vi "Write Enable Server Generic UE.vi"(10 "Enable Server Generic UE":bool, 11 "Template Server in":refnum<class "Streamer_server.lvclass">) -> (3 "Template Server out":refnum<class "Streamer_server.lvclass">)   [LabVIEW 2019, in "Streamer_server.lvlib" / "Streamer_server.lvclass"]
doc: "Enable the generic event if you would like to use a single event for capturing all messages. This would be useful if you are planning to implement your own dispatcher logic. \n\nKindly note that enabling the generic event would not generate the individual events."
uses:
  Streamer_server.lvclass
  Streamer_server.lvclass/Streamer_server.ctl
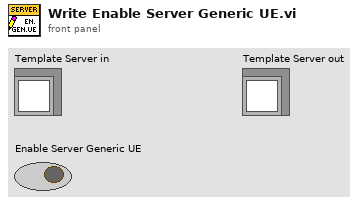
[diagram p1: front panel]
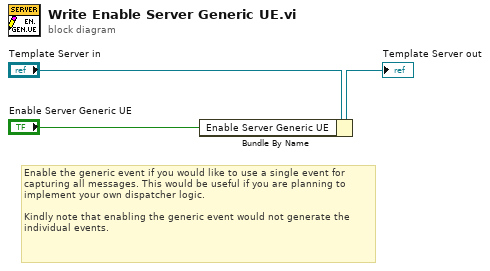
[diagram p0: block diagram]
diagram:
  # "Enable the generic event if you would like to use a single event for capturing all messages. This would be useful if you are planning to implement your own dispatcher logic. \n\nKindly note that enabling the generic event would not generate the individual events."
  n1 = Bundle By Name(cluster="Template Server in", "Enable Server Generic UE"="Enable Server Generic UE") -> (→"Template Server out":refnum<class "Streamer_server.lvclass">)
